vi "Destroy Client.vi"(8 "error in":errorcluster, 11 "gRPC ID":T1) -> (0 "error out":errorcluster)   [LabVIEW 2021, in "CIFTemplatePlugin_client.lvlib"]
uses:
  CIFTemplatePlugin_client.lvlib
  <vilib>/gRPC/LabVIEW gRPC Library/Shared/grpcId.ctl
  <vilib>/gRPC/LabVIEW gRPC Library/grpc-lvsupport-release.lvlib
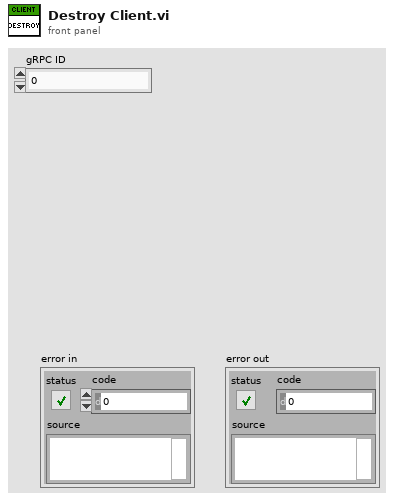
[diagram p1: front panel]
types:
  T1 = typedef "grpc-lvsupport-release.lvlib/grpcId.ctl" = u64
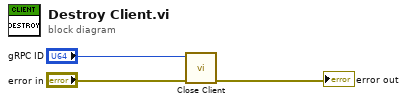
[diagram p0: block diagram]
diagram:
  n1 = call <vilib>:"Close Client.vi"("error in"="error in", "ClientID in"="gRPC ID") -> ("error out"=→"error out":errorcluster)  [unwired: 9 in]
